vi "Generate Scan Waveforms.vi"() -> ()   [LabVIEW 2018]
uses:
  <vilib>/Analysis/NI_AALBase.lvlib
  <vilib>/Analysis/1siggen.llb/Ramp Pattern by Samples.vi
  Controls/Translation Stage Types.ctl
  Hardware Mfg/Thorlabs Translation Stages/Controls/Translation Stage Cluster.ctl
  Controls/System Parameters.ctl
panel:
  in  "System Parameters [In]":T1={"Optical /HW Parameters"={"Focal Length [mm]"=0.0, "Scan Lens EFL[mm]"=0.0, "Tube Lens EFL[mm]"=0.0, "Galvo V Range (+/-)"=0.0, "Galvo Max Half Angle [Deg]"=0.0, "Max Galvo Range[%]"=0.0}, "Vibratome"={"Z Bottom [mm]"=0.0, "Pre Cut Dwell [s]"=0.0, "Blade Frequency [RPM]"=0, "Slice Speed [mm/s]"=0.0, "Post Cut Dwell [s]"=0.0, "Ramp Time [s]"=0.0, "Start X [mm]"=0.0, "Start Y [mm]"=0.0, "Slice Length [mm]"=0.0, "Slice Axis"=enum."Y Axis", "Controller VISA Ref"="COM4"}, "Table Stages"={"X Stage"={"Position"=0.0, "Is.Enabled?"=FALSE, "Is.Connected?"=FALSE, "Device SN"="45876539", "AccelerationMaximum"=0.0, "VelocityMaximum"=0.0, "Acceleration"=0.0, "Velocity"=0.0, "waitTimeout (ms)"=0, "Model"=enum."None", "Is.Homed?"=FALSE}, "Y Stage"={"Position"=0.0, "Is.Enabled?"=FALSE, "Is.Connected?"=FALSE, "Device SN"="45876539", "AccelerationMaximum"=0.0, "VelocityMaximum"=0.0, "Acceleration"=0.0, "Velocity"=0.0, "waitTimeout (ms)"=0, "Model"=enum."None", "Is.Homed?"=FALSE}, "Z Stage"={"Position"=0.0, "Is.Enabled?"=FALSE, "Is.Connected?"=FALSE, "Device SN"="45876539", "AccelerationMaximum"=0.0, "VelocityMaximum"=0.0, "Acceleration"=0.0, "Velocity"=0.0, "waitTimeout (ms)"=0, "Model"=enum."None", "Is.Homed?"=FALSE}}, "Imaging Parameter"={"Pixel Dwell Time"=0.0, "XY Center"={"Y"=1, "X"=1}, "Zoom Factor"=1, "Display Channel"=enum."Channel A", "XY Image Resolution"=enum."256 x 256", "Custom"=FALSE, "Averaging"={"A Frame Ave."=1, "B Frame Ave."=1, "C Frame Ave. "=1}}} {"Imaging Parameter"."XY Center"."Y" min=1 max=30 step=1; "Imaging Parameter"."XY Center"."X" min=1 max=30 step=1; "Imaging Parameter"."Averaging"."C Frame Ave." min=1 max=30 step=1; "Imaging Parameter"."Averaging"."B Frame Ave." min=1 max=30 step=1; "Imaging Parameter"."Averaging"."A Frame Ave." min=1 max=30 step=1; "Imaging Parameter"."Zoom Factor" min=1 max=10 step=1 scale=1.0..10.0; "Imaging Parameter"."Pixel Dwell Time" min=0.0 max=0.01 step=1e-05}
  # "X"
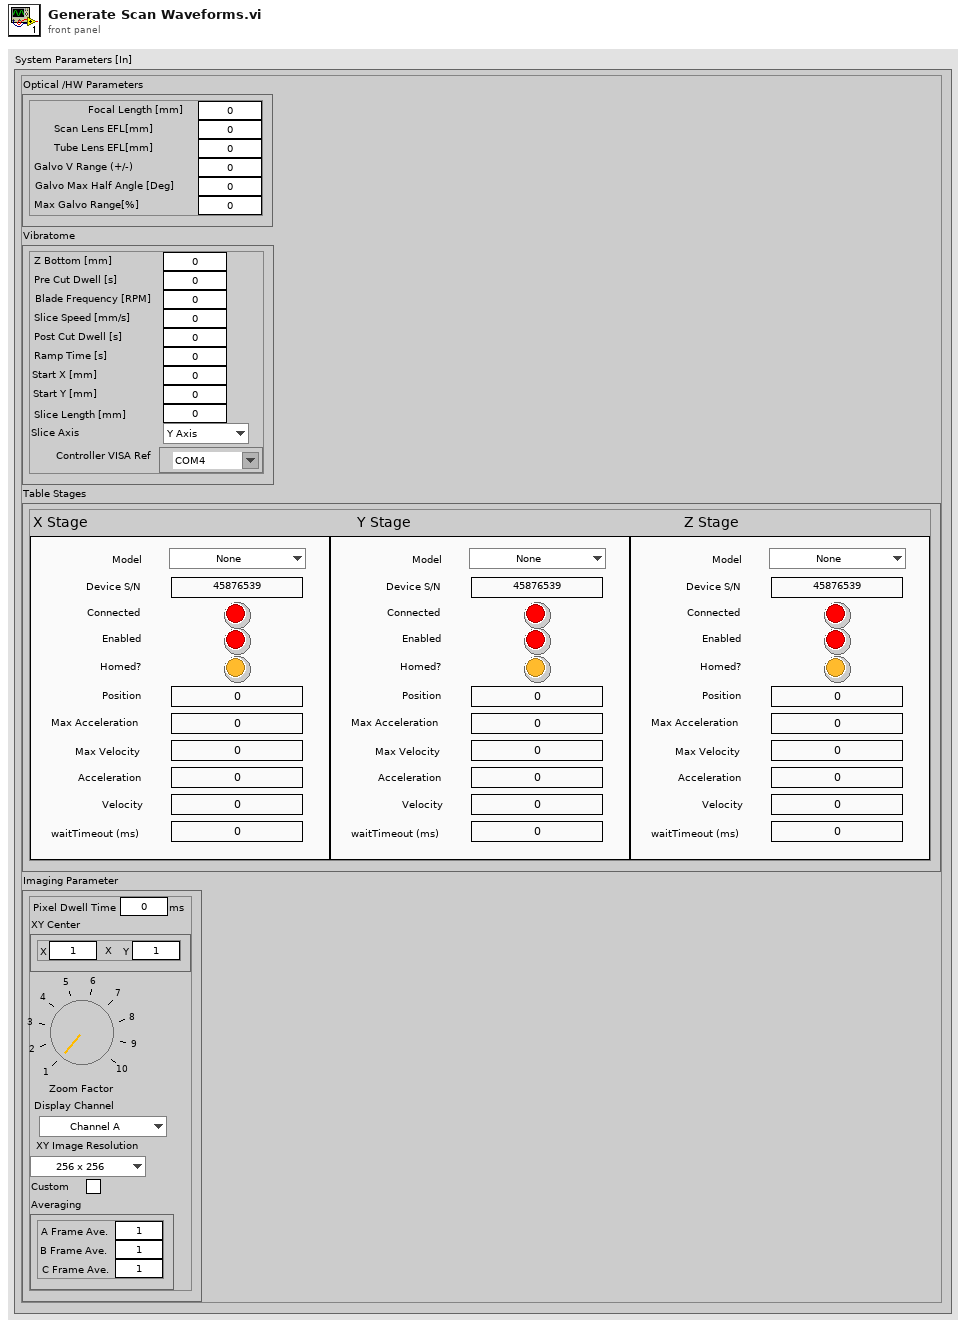
[diagram p1: front panel]
types:
  T1 = typedef "System Parameters.ctl" = cluster{"Optical /HW Parameters":cluster{"Focal Length [mm]":dbl[unit], "Scan Lens EFL[mm]":dbl[unit], "Tube Lens EFL[mm]":dbl[unit], "Galvo V Range (+/-)":dbl[unit], "Galvo Max Half Angle [Deg]":dbl[unit], "Max Galvo Range[%]":dbl[unit]}, "Vibratome":cluster{"Z Bottom [mm]":dbl, "Pre Cut Dwell [s]":dbl, "Blade Frequency [RPM]":u16, "Slice Speed [mm/s]":dbl, "Post Cut Dwell [s]":dbl, "Ramp Time [s]":dbl, "Start X [mm]":dbl, "Start Y [mm]":dbl, "Slice Length [mm]":dbl, "Slice Axis":enum16{"X Axis", "Y Axis", "Z Axis"}, "Controller VISA Ref":refnum<visa-resource-name>}, "Table Stages":cluster{"X Stage":T2, "Y Stage":T2, "Z Stage":T2}, "Imaging Parameter":cluster{"Pixel Dwell Time":dbl[unit], "XY Center":cluster{"Y":u16, "X":u16}, "Zoom Factor":u8, "Display Channel":enum16{"Channel A", "Channel B", "Channel A and B"}, "XY Image Resolution":enum16{"256 x 256", "512 x 512", "1024 x 1024", "2048 x 2048"}, "Custom":bool, "Averaging":cluster{"A Frame Ave.":u8, "B Frame Ave.":u8, "C Frame Ave. ":u8}}}
  T2 = typedef "Translation Stage Cluster.ctl" = cluster{"Position":dbl, "Is.Enabled?":bool, "Is.Connected?":bool, "Device SN":string, "AccelerationMaximum":dbl, "VelocityMaximum":dbl, "Acceleration":dbl, "Velocity":dbl, "waitTimeout (ms)":i32, "Model":T3, "Is.Homed?":bool}
  T3 = typedef "Translation Stage Types.ctl" = enum16{"None", "Thorlabs LTS", "Thorlabs MLJ"}
  T4 = cluster{"Focal Length [mm]":dbl[unit], "Scan Lens EFL[mm]":dbl[unit], "Tube Lens EFL[mm]":dbl[unit], "Galvo V Range (+/-)":dbl[unit], "Galvo Max Half Angle [Deg]":dbl[unit], "Max Galvo Range[%]":dbl[unit]}
  T5 = cluster{"Pixel Dwell Time":dbl[unit], "XY Center":cluster{"Y":u16, "X":u16}, "Zoom Factor":u8, "Display Channel":enum16{"Channel A", "Channel B", "Channel A and B"}, "XY Image Resolution":enum16{"256 x 256", "512 x 512", "1024 x 1024", "2048 x 2048"}, "Custom":bool, "Averaging":cluster{"A Frame Ave.":u8, "B Frame Ave.":u8, "C Frame Ave. ":u8}}
  T6 = enum16{"Channel A", "Channel B", "Channel A and B"}
  T7 = enum16{"256 x 256", "512 x 512", "1024 x 1024", "2048 x 2048"}
  T8 = cluster{"A Frame Ave.":u8, "B Frame Ave.":u8, "C Frame Ave. ":u8}
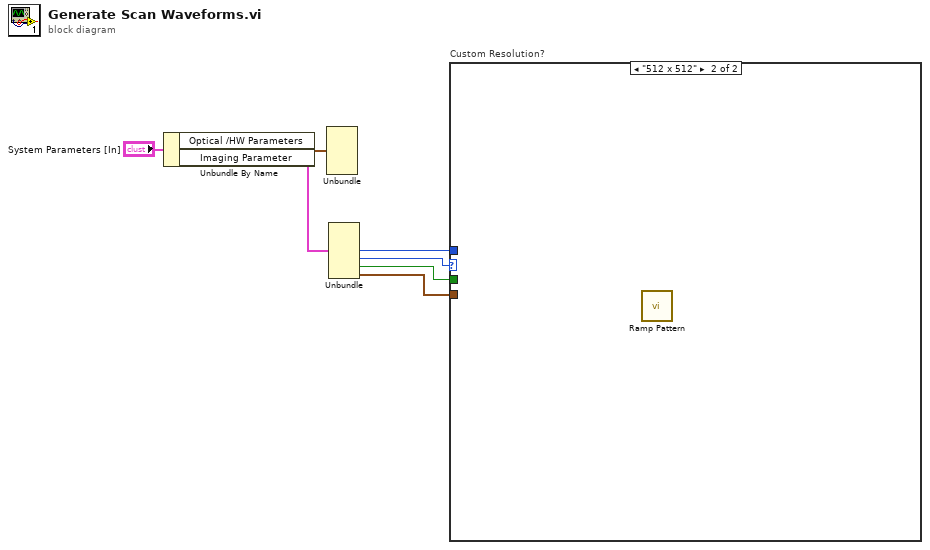
[diagram p0: block diagram]
diagram:
  n1 = Unbundle By Name("System Parameters [In]") -> ("Optical /HW Parameters"=w1:T4, "Imaging Parameter"=w6:T5)
  n2 = Unbundle(w1) -> ()  [unwired: 6 out]
  n3 = Unbundle(w6) -> ("Display Channel"=w4:T6, "XY Image Resolution"=w5:T7, "Custom"=w3:bool, "Averaging"=w2:T8)  [unwired: 3 out]
  n4 = case "Custom Resolution?" shown="\"512 x 512\"" w5 {
    tunnel: w4 -> [_ _]
    tunnel: w3 -> [_ _]
    tunnel: w2 -> [_ _]
    frame "256 x 256", Default {
    }
    frame "512 x 512" {
      n5 = call-poly <vilib>:"Ramp Pattern.vi"() -> ()  [unwired: 10 in, 2 out]
    }
  }
